vi "Merge Errors.vi"(2 "error in 2":errorcluster, 3 "error in":errorcluster) -> (0 "error out":errorcluster)   [LabVIEW 2015]
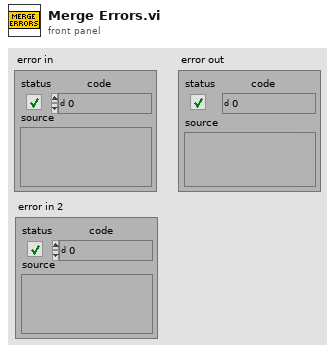
[diagram p1: front panel]
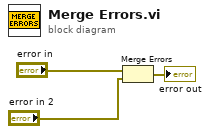
[diagram p0: block diagram]
diagram:
  n1 = Merge Errors("error in", "error in 2") -> (→"error out":errorcluster)
